vi "Edit Image Palette List Dialog.vi"(11 "Palette List (in)":string[](array[string])) -> (3 "Palette List (out)":string[](array[string]))   [LabVIEW 2021, in "Palette.lvlib"]
uses:
  Palette.lvlib
  <userlib>/_OpenG.lib/array/array.llb/Delete Elements from 1D Array (String)__ogtk.vi
  <userlib>/_OpenG.lib/array/array.llb/Sort 1D Array (String)__ogtk.vi
  <userlib>/_OpenG.lib/array/array.llb/openg_array.lvlib
panel:
  in  "OK":bool
  in  "Cancel":bool
  in  "Palette List":i32[](listbox)
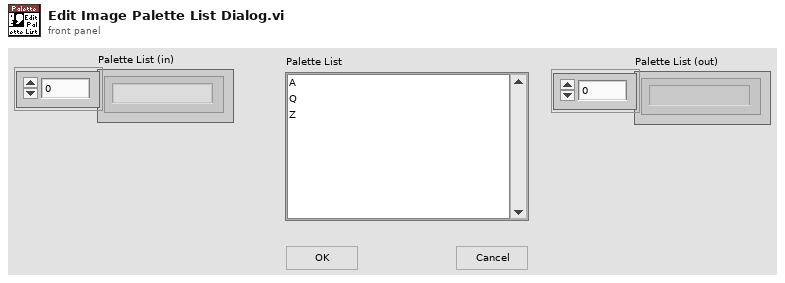
[diagram p1: front panel]
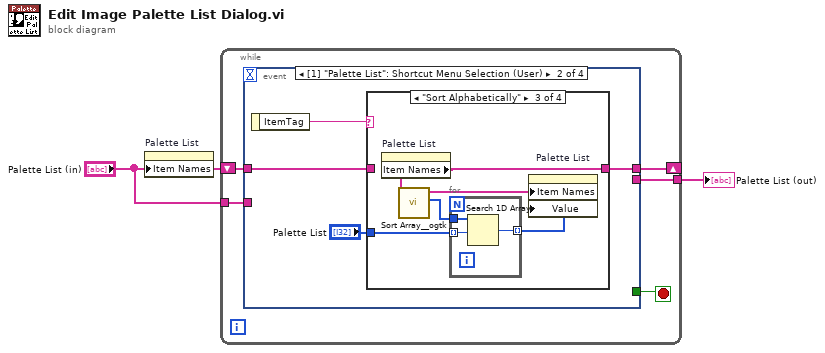
[diagram p0: block diagram]
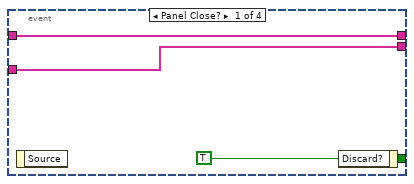
[diagram p2: hidden frame]
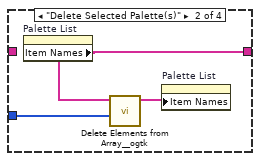
[diagram p4: hidden frame]
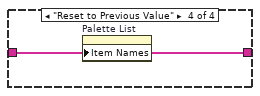
[diagram p5: hidden frame]
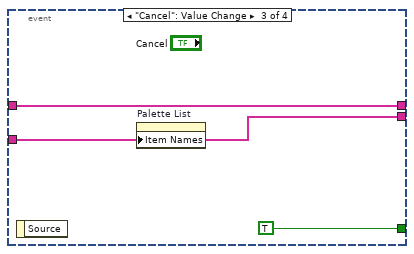
[diagram p6: hidden frame]
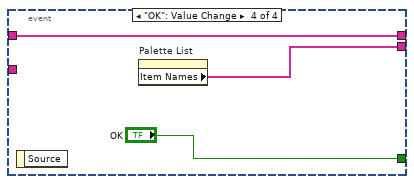
[diagram p7: hidden frame]
diagram:
  n1 = property on="Palette List" class="LstBox (strict)"("Item Names"="Palette List (in)") -> ()  [unwired: 2 in, 2 out]
  n2 = while {
    tunnel: "Palette List (in)" -> [w6]
    tunnel: [w5] -> w2
    shift-right: [w4] -> _
    shift-left: "Palette List (in)" -> [w3]
    stop <- w7 stop-if-true
    n3 = event shown="[1] \"Palette List\": Shortcut Menu Selection (User)" {
      selector: _ -> [_ _ _ _]
      dyn-events: _ -> [_ _ _ _]
      timeout: _ -> [_ _ _ _]
      tunnel: [w10 _ TRUE "OK"] -> w7
      tunnel: w6 -> [w9 _ w30 _]
      tunnel: [w9 _ w30 w33] -> w5
      tunnel: [w8 w12 w28 w31] -> w4
      tunnel: w3 -> [w8 w11 w28 w31]
      event Panel Close? {
        w10 = TRUE
        n4 = event-data() -> ()  [unwired: 1 in, 1 out]
        n5 = event-data("Discard?"=w10) -> ()  [unwired: 1 in, 1 out]
      }
      event "Palette List": Shortcut Menu Selection (User) {
        n6 = event-data() -> ("ItemTag"=w14:string)  [unwired: 1 in]
        n7 = case shown="\"Sort Alphabetically\"" w14 {
          tunnel: "Palette List" -> [_ w18 w21 _]
          tunnel: [w15 w16 w23 w27] -> w12
          tunnel: w11 -> [w15 _ _ w27]
          frame "", Default {
          }
          frame "Delete Selected Palette(s)" {
            n8 = property on="Palette List" class="LstBox (strict)"() -> ("Item Names"=w16:string[])  [unwired: 2 in, 2 out]
            n9 = call-poly <userlib>:"Delete Elements from Array__ogtk.vi"("indices"=w18, "array"=w16) -> ("array w/ subset deleted"=w17:string[])  [unwired: 8 in, 1 out]
            n10 = property on="Palette List" class="LstBox (strict)"("Item Names"=w17) -> ()  [unwired: 2 in, 2 out]
          }
          frame "Sort Alphabetically" {
            n11 = property on="Palette List" class="LstBox (strict)"() -> ("Item Names"=w23:string[])  [unwired: 2 in, 2 out]
            n12 = call-poly <userlib>:"Sort Array__ogtk.vi"("Array in"=w23) -> ("Sorted Pointers"=w20:i32[], "Sorted Array out"=w22:string[])  [unwired: 9 in]
            n13 = for {
              tunnel: w21 -> [w25] mode=indexing
              tunnel: w20 -> [w26]
              tunnel: [w24] -> w19 mode=indexing
              n14 = Search 1D Array(1D array=w26, element=w25) -> (index of element=w24:i32)  [unwired: 1 in]
            }
            n15 = property on="Palette List" class="LstBox (strict)"("Item Names"=w22, "Value"=w19) -> ()  [unwired: 2 in, 2 out]
          }
          frame "Reset to Previous Value" {
            n16 = property on="Palette List" class="LstBox (strict)"("Item Names"=w27) -> ()  [unwired: 2 in, 2 out]
          }
        }
      }
      event "Cancel": Value Change {
        n17 = event-data() -> ()  [unwired: 1 in, 1 out]
        n18 = property on="Palette List" class="LstBox (strict)"("Item Names"=w30) -> ()  [unwired: 2 in, 2 out]
      }
      event "OK": Value Change {
        n19 = event-data() -> ()  [unwired: 1 in, 1 out]
        n20 = property on="Palette List" class="LstBox (strict)"() -> ("Item Names"=w33:string[])  [unwired: 2 in, 2 out]
      }
    }
  }
  "Palette List (out)" <- w2
